vi "Quench detected.vi"() -> (0 "Stop":bool)   [LabVIEW 2019]
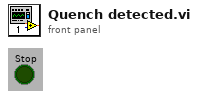
[diagram p1: front panel]
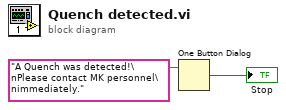
[diagram p0: block diagram]
diagram:
  n1 = One Button Dialog(message="A Quench was detected!\nPlease contact MK personnel\nimmediately.") -> (true=→"Stop":bool)  [unwired: 1 in]
